vi "Element Init.vi"(7 "VolatusAPI":refnum<class "VolatusAPI.lvclass">, 8 "error in (no error)":errorcluster, 10 "JSON":string, 11 "Control in":refnum<class "Control.lvclass">) -> (0 "error out":errorcluster, 3 "Control out":refnum<class "Control.lvclass">)   [LabVIEW 2020, in "VolatusGUI.lvlib" / "Control.lvclass"]
uses:
  Control.lvclass
  Volatus/VolatusAPI/VolatusAPI.lvclass
  Control.lvclass/Control.ctl
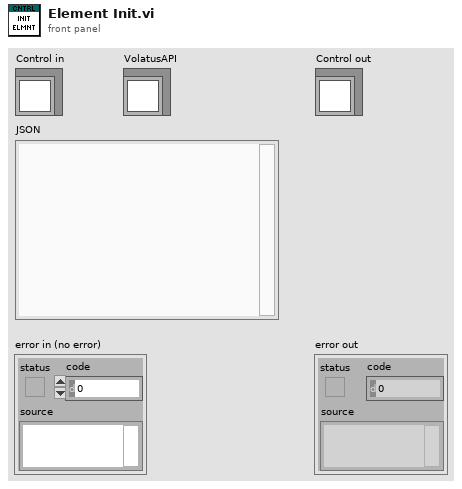
[diagram p1: front panel]
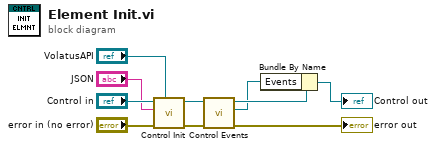
[diagram p0: block diagram]
diagram:
  n1 = call-dynamic "Control Init.vi"("VolatusAPI"="VolatusAPI", "error in (no error)"="error in (no error)", "JSON"="JSON", "Control in"="Control in") -> ("error out"=w9:errorcluster, "Control out"=w4:refnum<class "Control.lvclass">)  [unwired: 6 in]
  n2 = call-dynamic "Control Events.vi"("error in (no error)"=w9, "Control in"=w4) -> ("error out"=→"error out":errorcluster, "Control Events"=w1:refnum<class "Control Event Registrations.lvclass">, "Control out"=w3:refnum<class "Control.lvclass">)  [unwired: 7 in]
  n3 = Bundle By Name(cluster=w3, "Events"=w1) -> (→"Control out":refnum<class "Control.lvclass">)
